vi "Apply Default Name.vi"(8 "error in (no error)":errorcluster, 11 "Step in":refnum<class "Step.lvclass">) -> (0 "error out":errorcluster, 3 "Step out":refnum<class "Step.lvclass">)   [LabVIEW 2020, in "TSnax.lvlib" / "Step.lvclass"]
uses:
  Step.lvclass
  C:/dev/illuminated-g/tsnax/TSnax/PropertyObject/PropertyObject.lvclass
  67d219c6-c51a-4e80-b631-31afe947a0fd.vi/cb391dcb-11b9-4fdf-8aeb-34376e1cbb94.vi
  67d219c6-c51a-4e80-b631-31afe947a0fd.vi/d46dfaf5-493f-4f70-8e7b-742c39259470.vi
  67d219c6-c51a-4e80-b631-31afe947a0fd.vi/d46dfaf5-493f-4f70-8e7b-742c39259470.vi/5752542f-8fd2-4c21-a269-ab70273be737.vi
  PropertyObject/Get Val STR.vi
  PropertyObject/Eval Expression String.vi
  PropertyObject/PropertyObject.lvclass
  Step.lvclass/Step.ctl
  00368093-8b12-4d85-ae91-f0b0dbe370d0.vi
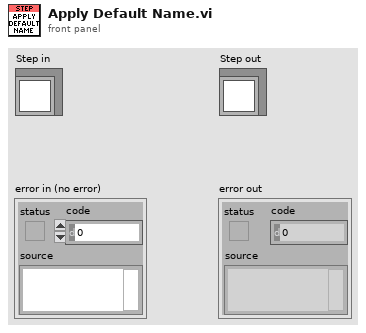
[diagram p1: front panel]
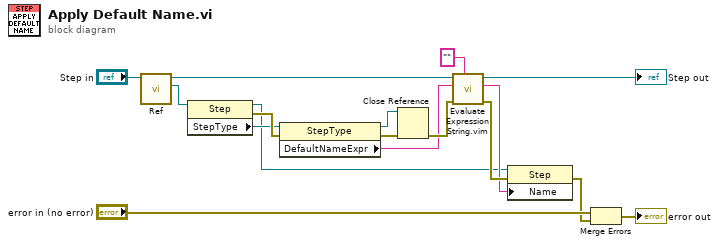
[diagram p0: block diagram]
diagram:
  n1 = call "Ref.vi"("Step in"="Step in") -> ("Step"=w12:refnum<k7>, "Step out"=w9:refnum<class "Step.lvclass">)  [unwired: 8 in, 1 out]
  n2 = property class="Step"(reference=w12) -> (reference out=w1:refnum<k7>, error out=w17:errorcluster, "StepType"=w4:refnum<k7>)  [unwired: 1 in]
  n3 = property class="StepType"(reference=w4, error in=w17) -> (reference out=w10:refnum<k7>, error out=w11:errorcluster, "DefaultNameExpr"=w7:string)
  n4 = Close Reference(reference=w10, error in (no error)=w11) -> (error out=w8:errorcluster)
  n5 = call "Evaluate Expression String.vim"("Result Type (PropertyObject)"="", "error in (no error)"=w8, "Expression String"=w7, "PropertyObject in"=w9) -> ("error out"=w6:errorcluster, "Result"=w3:string, "PropertyObject out"=→"Step out":refnum<class "Step.lvclass">)  [unwired: 5 in]
  n6 = property class="Step"(reference=w1, error in=w6, "Name"=w3) -> (error out=w14:errorcluster)  [unwired: 1 out]
  n7 = Merge Errors("error in (no error)", w14) -> (→"error out":errorcluster)
